vi "Mixer.Write Level.vi"(0 "baseURL":string="http://169.254.128.32/datastore/", 7 "value":dbl, 11 "error in (no error)":errorcluster) -> (4 "baseURL out":string="http://169.254.128.32/datastore/", 15 "error out":errorcluster)   [LabVIEW 2020]
uses:
  <vilib>/httpClient/POSTBuffer.vi
  <vilib>/httpClient/LabVIEWHTTPClient.lvlib
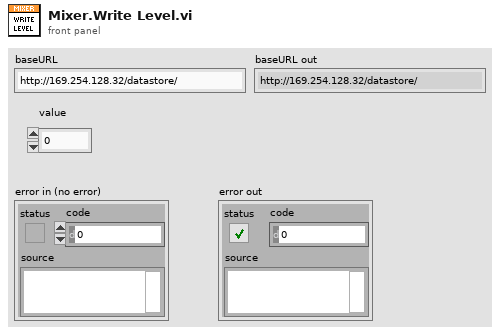
[diagram p1: front panel]
types:
  T1 = typedef "LabVIEWHTTPClient.lvlib/ClientHandle.ctl" = refnum<k1>
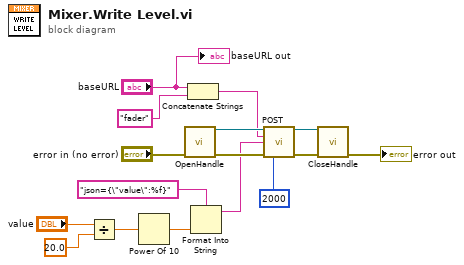
[diagram p0: block diagram]
diagram:
  n1 = Divide(x="value", y=20.0) -> (x/y=w3:dbl)
  n2 = Power Of 10(x=w3) -> (10^x=w2:dbl)
  n3 = call <vilib>:"OpenHandle.vi"("error in (no error)"="error in (no error)") -> ("client handle out"=w13:T1, "error out"=w12:errorcluster)  [unwired: 13 in]
  n4 = Concatenate Strings("baseURL", "fader") -> (w11:string)
  n5 = Format Into String(format string="json={\"value\":%f}" ("buffer"), w2) -> (resulting string=w7:string)  [unwired: 2 in, 1 out]
  n6 = call-poly <vilib>:"POST.vi"("client handle"=w13, "url"=w11, "buffer"=w7, "error in (no error)"=w12, "timeout (10000)"=2000) -> ("client handle out"=w15:T1, "error out"=w16:errorcluster)  [unwired: 7 in, 2 out]
  n7 = call <vilib>:"CloseHandle.vi"("client handle"=w15, "error in (no error)"=w16) -> ("error out"=→"error out":errorcluster)  [unwired: 13 in]
  "baseURL out" <- "baseURL"
